vi "QSM_Wait on Dequeue.vi"(0 "QSM_ShiftRegister in":T2 {"ROI Process"."Particle Variables" items=["Center of Mass X", "Center of Mass Y", "First Pixel X", "First Pixel Y", "Bounding Rect Left", "Bounding Rect Top", "Bounding Rect Right", "Bounding Rect Bottom", "Max Feret Diameter Start X", "Max Feret Diameter Start Y", "Max Feret Diameter End X", "Max Feret Diameter End Y", "Max Horiz. Segment Length Left", "Max Horiz. Segment Length Right", "Max Horiz. Segment Length Row", "-", "Bounding Rect Width", "Bounding Rect Height", "Bounding Rect Diagonal", "Perimeter", "Convex Hull Perimeter", "Holes' Perimeter", "Max Feret Diameter", "Equivalent Ellipse Major Axis", "Equivalent Ellipse Minor Axis", "Equivalent Ellipse Minor Axis (Feret)", "Equivalent Rect Long Side", "Equivalent Rect Short Side", "Equivalent Rect Diagonal", "Equivalent Rect Short Side (Feret)", "Average Horiz. Segment Length", "Average Vert. Segment Length", "Hydraulic Radius", "Waddel Disk Diameter", "-", "Area", "Holes' Area", "Particle & Holes' Area", "Convex Hull Area", "Image Area", "-", "Number of Holes", "Number of Horiz. Segments", "Number of Vert. Segments", "-", "Orientation", "Max Feret Diameter Orientation", "-", "% Area/Image Area", "% Area/(Particle & Holes' Area)", "Ratio of Equivalent Ellipse Axes", "Ratio of Equivalent Rect Sides", "-", "Elongation Factor", "Compactness Factor", "Heywood Circularity Factor", "Type Factor", "-", "Sum X", "Sum Y", "Sum XX", "Sum XY", "Sum YY", "Sum XXX", "Sum XXY", "Sum XYY", "Sum YYY", "-", "Moment of Inertia XX", "Moment of Inertia XY", "Moment of Inertia YY", "Moment of Inertia XXX", "Moment of Inertia XXY", "Moment of Inertia XYY", "Moment of Inertia YYY", "Norm. Moment of Inertia XX", "Norm. Moment of Inertia XY", "Norm. Moment of Inertia YY", "Norm. Moment of Inertia XXX", "Norm. Moment of Inertia XXY", "Norm. Moment of Inertia XYY", "Norm. Moment of Inertia YYY", "Hu Moment 1", "Hu Moment 2", "Hu Moment 3", "Hu Moment 4", "Hu Moment 5", "Hu Moment 6", "Hu Moment 7"]; "ROI Process"."Particle Measurements (Pixels)" format="%.2f"; "ROI Process"."ROIS"."Contours"."Type" items=["No Selection", "Point", "Line", "Rectangle", "Oval", "Polygon", "Freehand Region", "Annulus", "Unused2", "Unused3", "Broken Line", "Freehand Line", "Rotated Rectangle"]; "Single Image Results"."ROI Results"."LIMLOCALMETADATA"."dTimeMSec" format="%.2f"}, 5 "timeout in ms (-1)":i32=-1, 11 "error in (no error)":errorcluster) -> (4 "Queue References.QSMRef out":T5, 6 "RunStates_TEST":T1, 8 "DATA.VARIANT":variant, 10 "timed out?":bool, 15 "error out":errorcluster)   [LabVIEW 2014, in "TestQSM.lvlib"]
uses:
  TestQSM.lvlib
  Controls/QSM_Reference.ctl
  Controls/QSM_DataType.ctl
  Controls/QSM_RunStates.ctl
  Controls/QSM_ShiftRegister.ctl
  QueueMaintenance/TypeDef/QSMRef_ALL.ctl
  Queue_TESTGUIUPDATE/Controls/QSM_Reference.ctl
  Queue_TESTGUIUPDATE/Controls/QSM_DataType.ctl
  Queue_TESTGUIUPDATE/Controls/QSM_RunStates.ctl
  Custom Controls/cluster - Image Results.ctl
  ND2_Reader_32bit/controls/cluster_LIMLOCALMETADATA.ctl
  Queue_TESTGUIUPDATE/GUIUpdateQSM.lvlib
  QueueMaintenance/QueueMaintenance.lvlib
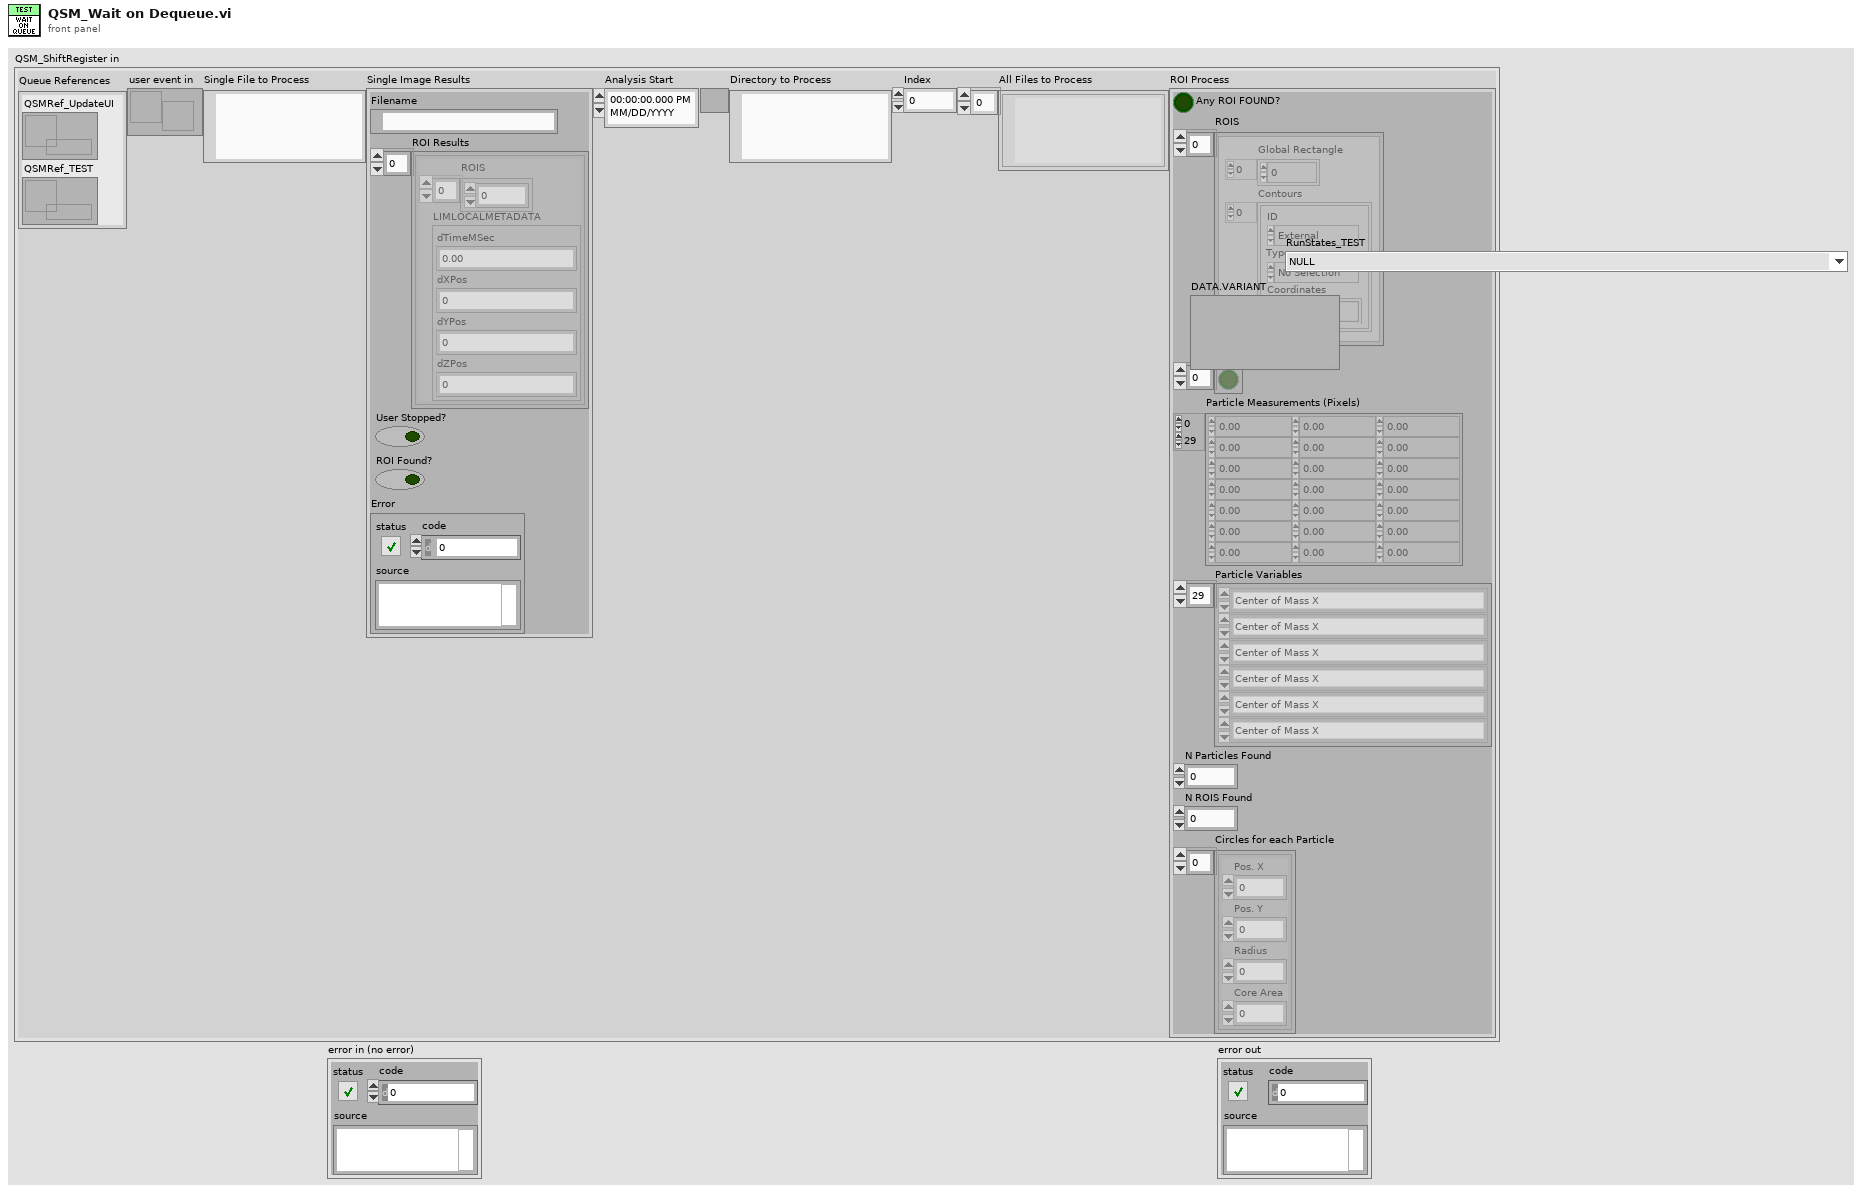
[diagram p1: front panel]
types:
  T1 = typedef "TestQSM.lvlib/QSM_RunStates.ctl" = enum16{"NULL", "Sect01-Initialize-00-GROUP.ENQUEUE", "Sect02-Single File_Check for Parameters", "Sect02-Single File_Ask for File", "Sect02-Single File_Run Analysis", "Sect02-Single File_Write Results", "Sect03-Single ROI Calc_Check for Parameters", "Sect03-Single ROI Calc_Ask for File", "Sect03-Single ROI Calc_Run Analysis", "Sect03-Single ROI _Write Results", "Sect12-Full Dir_Check for Parameters", "Sect12-Full Dir_Ask for Dir", "Sect12-Full Dir_Check for Next Image to Process", "Sect12-Full Dir_Run Analysis", "Sect12-Full Dir_Write Results", "Sect12-Full Dir_Check if User Stopped", "Sect13-FullDir ROI Calc_Check for Parameters", "Sect13-FullDir ROI Calc_Ask for Dir", "Sect13-Full Dir ROI Calc_Check for Next Image to Process", "Sect13-Full Dir ROI Calc_Run Analysis", "Sect13-Full Dir ROI Calc_Write Results", "Sect13-Full Dir ROI Calc_Check if User Stopped", "Sect90-GUI_Config_Change UI Before Analysis", "Sect90-GUI_Config_Change UI After Analysis", "Sect90-GUI_Stop Processing Pressed", "Sect90-GUI_Stop Processing Button Set Back to F", "Sect90-GUI_Clear ROIs", "Sect99_EXIT-00-Group.Enqueue", "Sect99_EXIT-01-StopQSM"}
  T2 = typedef "TestQSM.lvlib/QSM_ShiftRegister.ctl" = cluster{"Queue References":T3, "user event in":refnum<user-event>, "Single File to Process":path, "Single Image Results":T6, "Analysis Start":timestamp, "Directory to Process":path, "Index":i32, "All Files to Process":path[], "ROI Process":cluster{"Any ROI FOUND?":bool, "ROIS":T8[], "ROIS Found?":bool[], "Particle Measurements (Pixels)":dbl[][], "Particle Variables":i32[], "N Particles Found":i32, "N ROIS Found":i32, "Circles for each Particle":cluster{"Pos. X":i32, "Pos. Y":i32, "Radius":i32, "Core Area":i32}[]}}
  T3 = typedef "QueueMaintenance.lvlib/QSMRef_ALL.ctl" = cluster{"QSMRef_UpdateUI":T4, "QSMRef_TEST":T5}
  T4 = typedef "GUIUpdateQSM.lvlib/QSM_Reference.ctl" = refnum<queue>
  T5 = typedef "TestQSM.lvlib/QSM_Reference.ctl" = refnum<queue>
  T6 = typedef "cluster - Image Results.ctl" = cluster{"Filename":path, "ROI Results":cluster{"ROIS":dbl[], "LIMLOCALMETADATA":T7}[], "User Stopped?":bool, "ROI Found?":bool, "Error":errorcluster}
  T7 = typedef "cluster_LIMLOCALMETADATA.ctl" = cluster{"dTimeMSec":dbl, "dXPos":dbl, "dYPos":dbl, "dZPos":dbl}
  T8 = typedef "ROI Descriptor" = cluster{"Global Rectangle":i32[], "Contours":cluster{"ID":enum32{"External", "Internal"}, "Type":u32, "Coordinates":i32[]}[]}
  T9 = typedef "TestQSM.lvlib/QSM_DataType.ctl" = cluster{"RunStates":T1, "Data (Variant)":variant}
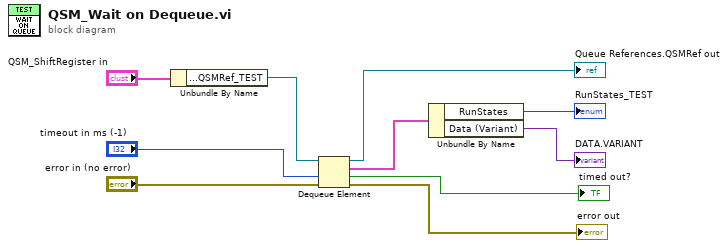
[diagram p0: block diagram]
diagram:
  n1 = Unbundle By Name("QSM_ShiftRegister in") -> ("Queue References.QSMRef_TEST"=w6:T5)
  n2 = Dequeue Element(queue=w6, timeout in ms (-1)="timeout in ms (-1)", error in (no error)="error in (no error)") -> (queue out=→"Queue References.QSMRef out":T5, element=w4:T9, timed out?=→"timed out?":bool, error out=→"error out":errorcluster)
  n3 = Unbundle By Name(w4) -> ("RunStates"=→"RunStates_TEST":T1, "Data (Variant)"=→"DATA.VARIANT":variant)
